vi "Control_ReadJoystick4.vi"() -> (4 "Up":bool, 6 "Down":bool, 8 "Left":bool, 10 "Right":bool, 15 "Button":bool)   [LabVIEW 2018]
uses:
  <vilib>/rvi/eio/common/nirviEmuTemplateMethod_errors.vi
  <vilib>/eio/EIONode/EIONode.xnode
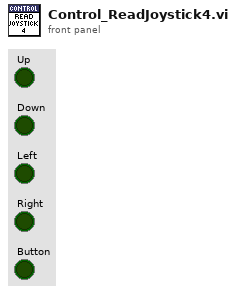
[diagram p1: front panel]
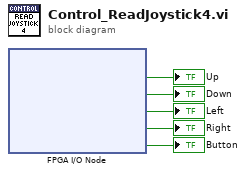
[diagram p0: block diagram]
diagram:
  n1 = xnode "FPGA I/O Node"() -> ("ConnectorB/DIO5"=→"Up":bool, "ConnectorB/DIO6"=→"Down":bool, "ConnectorB/DIO7"=→"Left":bool, "ConnectorB/DIO8"=→"Right":bool, "ConnectorB/DIO9"=→"Button":bool)  [unwired: 5 in, 5 out]
